vi "command update firmware.vi"(8 "error in (no error)":errorcluster, 9 "data_size":u32, 10 "data":u8, 11 "name":string) -> (0 "error out":errorcluster, 3 "function return":i32)   [LabVIEW 2012, in "libximc.lvlib"]
doc: "result_t XIMC_API command_update_firmware(const char* name, const uint8_t* data, uint32_t data_size);"
uses:
  libximc.lvlib
  libximc.dll
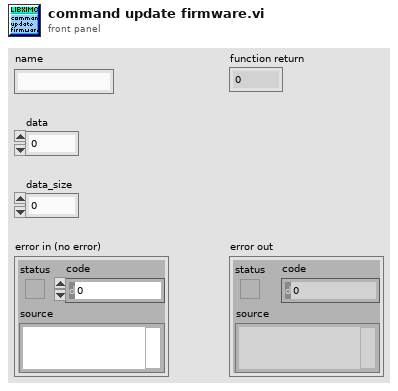
[diagram p1: front panel]
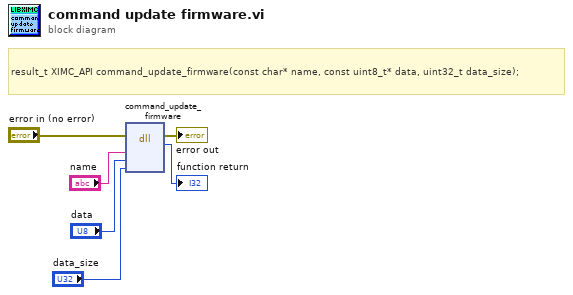
[diagram p0: block diagram]
diagram:
  # "result_t XIMC_API command_update_firmware(const char* name, const uint8_t* data, uint32_t data_size);"
  n1 = dll-call lib="C:/Users/Stepan/Downloads/labview_2.9.11_testgen_thread/libximc.*" fn="command_update_firmware"(error in="error in (no error)", "name"="name", "data"="data", "data_size"="data_size") -> (error out=→"error out":errorcluster, →"function return":i32)  [unwired: 5 in, 1 out]
